vi "data between cursors.vi"(0 "cursor 1 X":dbl, 1 "cursor 2 X":dbl, 3 "Curve fit all data":bool, 5 "X in":i32[](array[numeric]), 9 "Y in":i32[](array[numeric]), 11 "index start in":i32, 12 "array length in":i32, 14 "first case date":timestamp) -> (4 "X out":i32[](array[numeric]), 6 "Y out":i32[](array[numeric]), 10 "index start out":i32, 15 "array length out":i32)   [LabVIEW 2019]
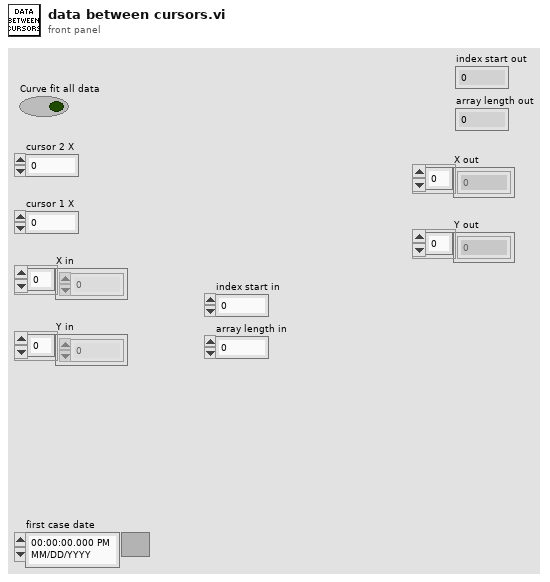
[diagram p1: front panel]
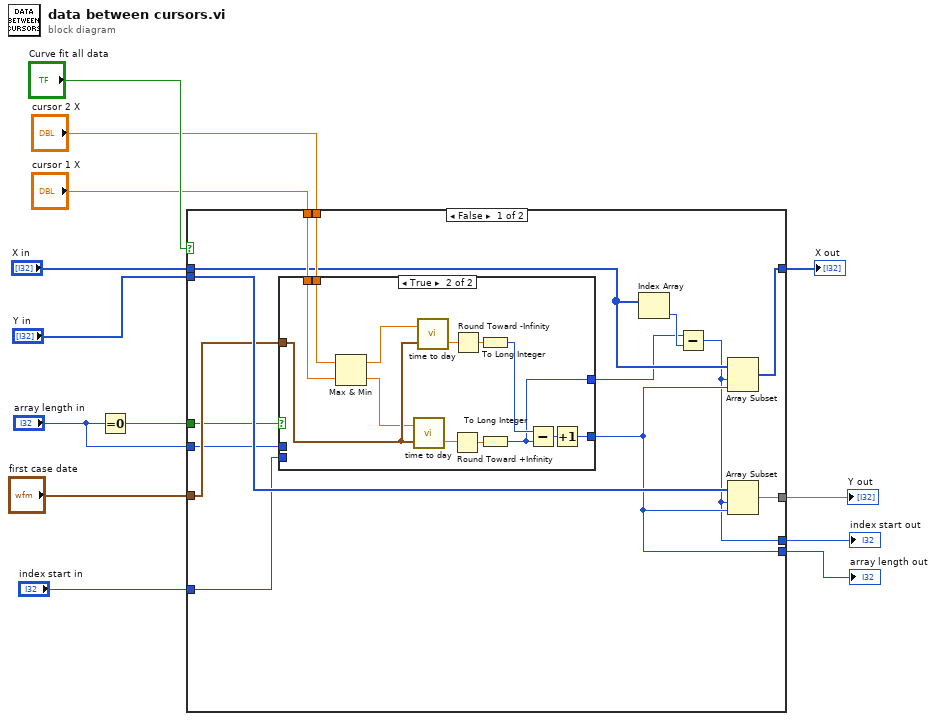
[diagram p0: block diagram]
diagram:
  n1 = Equal To 0?(x="array length in") -> (x = 0?=w3:bool)
  n2 = case shown="False" "Curve fit all data" {
    tunnel: "X in" -> [w17 w46]
    tunnel: "Y in" -> [w26 w45]
    tunnel: [w27 w46] -> w8
    tunnel: [w25 w45] -> w9
    tunnel: "first case date" -> [w24 _]
    tunnel: "cursor 2 X" -> [w23 _]
    tunnel: "cursor 1 X" -> [w22 _]
    tunnel: [w15 w44] -> w5
    tunnel: [w21 w43] -> w4
    tunnel: w3 -> [w20 _]
    tunnel: "array length in" -> [w19 w43]
    tunnel: "index start in" -> [w18 w44]
    frame False {
      n3 = case shown="True" w20 {
        tunnel: w24 -> [_ w42]
        tunnel: w23 -> [_ w41]
        tunnel: w22 -> [_ w40]
        tunnel: [w29 w34] -> w14
        tunnel: [w28 w30] -> w21
        tunnel: w19 -> [w28 _]
        tunnel: w18 -> [w29 _]
        frame False {
        }
        frame True {
          n4 = Max & Min(x=w41, y=w40) -> (max(x,y)=w33:dbl, min(x,y)=w32:dbl)
          n5 = call "time to day.vi"("time offset"=w42, "time in seconds"=w32) -> ("fractional day"=w36:dbl)  [unwired: 1 out]
          n6 = call "time to day.vi"("time offset"=w42, "time in seconds"=w33) -> ("fractional day"=w39:dbl)  [unwired: 1 out]
          n7 = Round Toward +Infinity(x=w36) -> (ceil(x): smallest int >= x=w35:dbl)
          n8 = Round Toward -Infinity(1:w39) -> (0:w38:dbl)
          n9 = To Long Integer(number=w38) -> (32bit integer=w37:i32)
          n10 = To Long Integer(number=w35) -> (32bit integer=w34:i32)
          n11 = Subtract(x=w37, y=w34) -> (x-y=w31:i32)
          n12 = Increment(x=w31) -> (x+1=w30:i32)
        }
      }
      n13 = Index Array(array=w17) -> (element=w16:i32)  [unwired: 1 in]
      n14 = Subtract(x=w14, y=w16) -> (x-y=w15:i32)
      n15 = Array Subset(array=w17, index=w15, length=w21) -> (w27:i32[])
      n16 = Array Subset(array=w26, index=w15, length=w21) -> (w25:i32[])
    }
    frame True {
    }
  }
  "Y out" <- w9
  "X out" <- w8
  "index start out" <- w5
  "array length out" <- w4
